vi "Data Sender.vi"() -> ()   [LabVIEW 2018]
uses:
  <vilib>/userdefined/High Color/IMAQdx.ctl
  <vilib>/DAQmx/read.llb/DAQmx Read (Analog 2D DBL NChan NSamp).vi
  <vilib>/DAQmx/miscellaneous.llb/DAQmx Fill In Error Info.vi
  <vilib>/vision/driver/NI_Vision_Acquisition_Software.lvlib
panel:
  in  "Stop 2":bool
  in  "Save Binary":bool
  in  "Save AVI":bool
  out "Image 3":T1(plugin-control)
  in  "Image Type":T2 items=["Grayscale (U8)", "Grayscale (I16)", "Grayscale (SGL)", "Complex (CSG)", "RGB (U32)", "HSL (U32)", "RGB (U64)", "Grayscale (U16)"]
  out "Frame Number Recorded":i32
  in  "number":i32
  in  "File Folder":path
  in  "Video Camera":T3 caption="Camera Name"
  # "Binary Video"
  # "AVI Video"
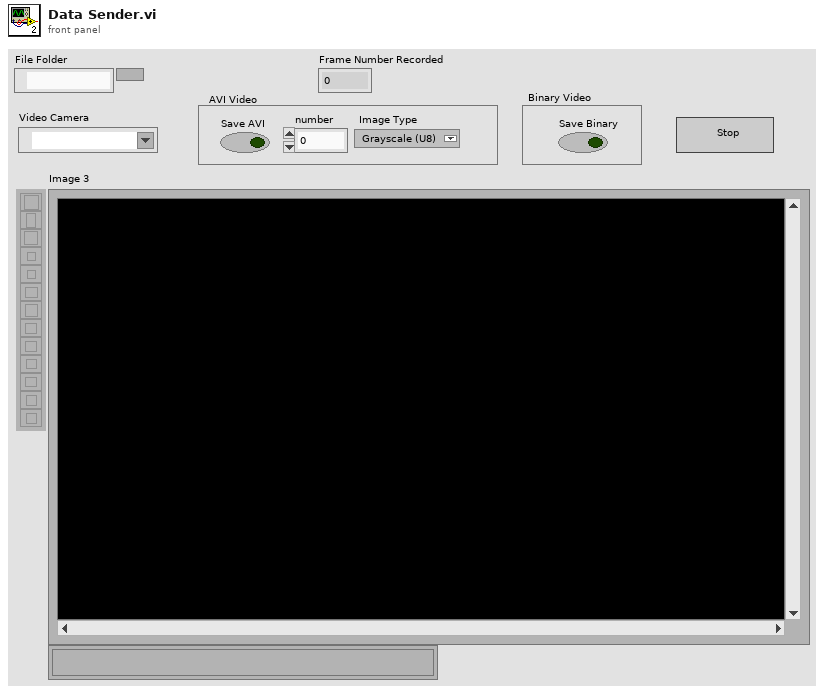
[diagram p1: front panel]
types:
  T1 = typedef "IMAQ Image.ctl" = refnum<image>
  T2 = typedef "Image Type" = u32
  T3 = typedef "IMAQdx.ctl" = refnum<k21>
  T4 = typedef "IMAQ AVI2 Refnum.ctl" = refnum<k20>
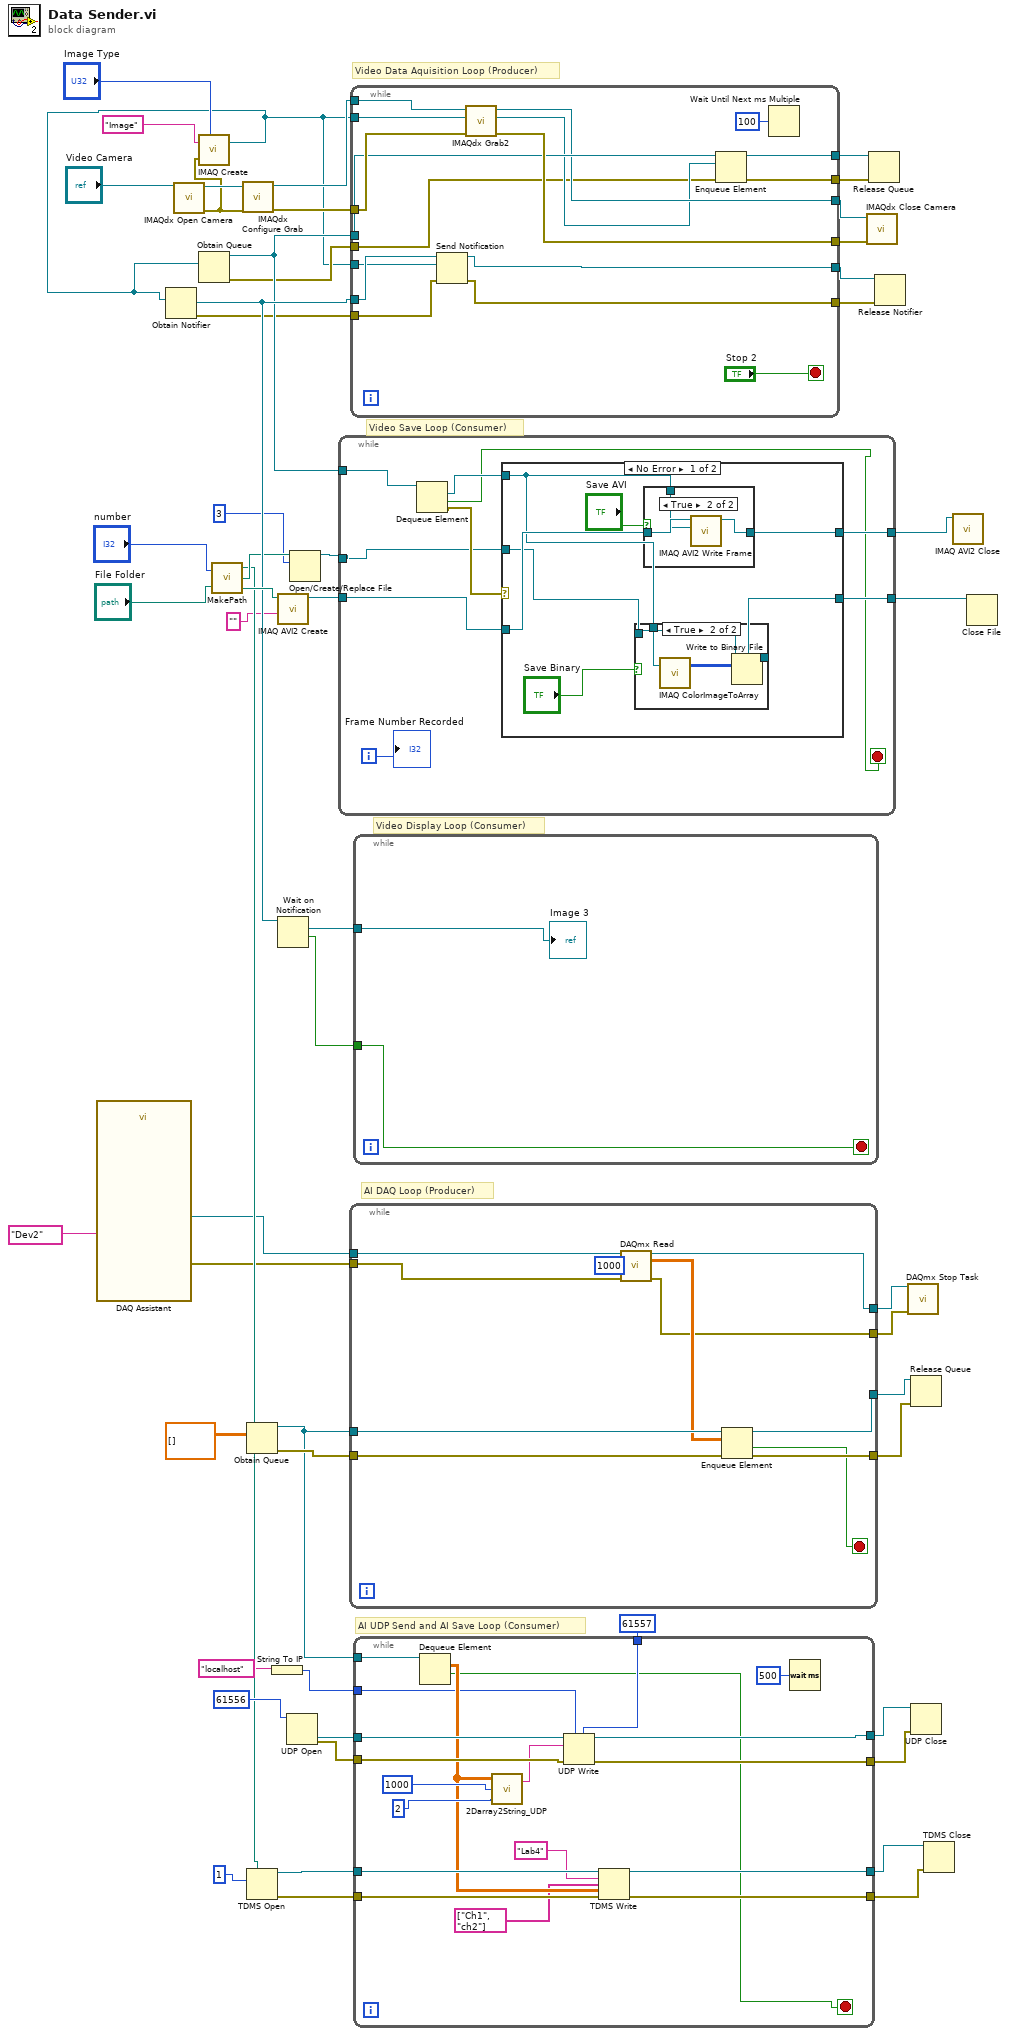
[diagram p0: block diagram]
diagram:
  # "AI UDP Send and AI Save Loop (Consumer)"
  # "AI DAQ Loop (Producer)"
  # "Video Display Loop (Consumer)"
  # "Video Save Loop (Consumer)"
  # "Video Data Aquisition Loop (Producer)"
  n1 = call "DAQ Assistant"("device name"=tag "Dev2") -> ("task out"=w7:refnum<k21>, "error out"=w6:errorcluster)  [unwired: 15 in, 2 out]
  n2 = call <vilib>:"IMAQdx Open Camera.vi"("Session In"="Video Camera") -> ("error out"=w45:errorcluster, "Session Out"=w53:T3)  [unwired: 9 in]
  n3 = call "IMAQ Create"("Image Name"="Image", "Image Type"="Image Type", "error in (no error)"=w45) -> ("New Image"=w27:T1)  [unwired: 2 in, 1 out]
  n4 = Obtain Notifier(notification data type=w27) -> (notifier out=w40:refnum<notifier>, error out=w32:errorcluster)  [unwired: 3 in, 1 out]
  n5 = Obtain Queue(element data type=w27) -> (queue out=w38:refnum<queue>, error out=w30:errorcluster)  [unwired: 4 in, 1 out]
  n6 = call "MakePath.vi"("Numeric"="number", "Path"="File Folder") -> ("TDMS"=w8:path, "BIN"=w35:path, "AVI"=w44:path)
  n7 = call <vilib>:"IMAQdx Configure Grab.vi"("error in"=w45, "Session In"=w53) -> ("error out"=w52:errorcluster, "Session Out"=w33:T3)  [unwired: 8 in]
  n8 = Obtain Queue(element data type=dbl[][] [] ("data")) -> (queue out=w11:refnum<queue>, error out=w22:errorcluster)  [unwired: 4 in, 1 out]
  n9 = TDMS Open(10:1, 11:w8) -> (0:w15:errorcluster, 3:w16:refnum<k34>)  [unwired: 5 in]
  n10 = String To IP(1:"localhost") -> (0:w2:u32)
  n11 = call "IMAQ AVI2 Create"("Codec"="", "AVI Path"=w44) -> ("AVI Refnum"=w43:T4)  [unwired: 8 in, 1 out]
  n12 = Wait on Notification(notifier=w40) -> (notification=w39:T1, timed out?=w9:bool)  [unwired: 3 in, 2 out]
  n13 = UDP Open(11:61556) -> (port=w20:refnum<k16>, 0:w21:errorcluster)  [unwired: 4 in, 1 out]
  n14 = Open/Create/Replace File(file path (use dialog)=w35, operation (0:open)=3) -> (refnum out=w36:refnum<file>)  [unwired: 4 in, 2 out]
  n15 = while {
    tunnel: w43 -> [w60]
    tunnel: w36 -> [w61]
    tunnel: [w59] -> w42
    tunnel: [w58] -> w41
    tunnel: w38 -> [w57]
    i -> [w62]
    stop <- w55 stop-if-true
    n16 = Dequeue Element(queue=w57) -> (element=w56:T1, timed out?=w55:bool, error out=w63:errorcluster)  [unwired: 2 in, 1 out]
    n17 = case shown="No Error" w63 {
      tunnel: w61 -> [w69 w80]
      tunnel: w60 -> [w70 w81]
      tunnel: [w68 w81] -> w59
      tunnel: [w67 w80] -> w58
      tunnel: w56 -> [w66 _]
      frame No Error {
        n18 = case shown="True" "Save Binary" {
          tunnel: w69 -> [w71 w75]
          tunnel: [w71 w74] -> w67
          tunnel: w66 -> [_ w73]
          frame False {
          }
          frame True {
            n19 = call "IMAQ ColorImageToArray"("Image"=w73) -> ("Image Pixels (U32)"=w72:u32[][])  [unwired: 3 in, 2 out]
            n20 = Write to Binary File(file (use dialog)=w75, data=w72) -> (refnum out=w74:refnum<file>)  [unwired: 4 in, 2 out]
          }
        }
        n21 = case shown="True" "Save AVI" {
          tunnel: w70 -> [w76 w79]
          tunnel: [w76 w78] -> w68
          tunnel: w66 -> [_ w77]
          frame False {
          }
          frame True {
            n22 = call "IMAQ AVI2 Write Frame"("Image"=w77, "AVI Refnum"=w79) -> ("AVI Refnum (duplicate)"=w78:T4)  [unwired: 7 in, 2 out]
          }
        }
      }
      frame Error {
      }
    }
    "Frame Number Recorded" <- w62
  }
  n23 = while {
    tunnel: w11 -> [w92]
    tunnel: [w86] -> w26
    tunnel: [w87] -> w25
    tunnel: [w91] -> w24
    tunnel: [w90] -> w23
    tunnel: w22 -> [w89]
    tunnel: w7 -> [w83]
    tunnel: w6 -> [w82]
    stop <- w85 stop-if-true
    n24 = call-poly <vilib>:"DAQmx Read.vi"("task/channels in"=w83, "number of samples per channel"=1000, "error in"=w82) -> ("task out"=w86:refnum<k21>, "data"=w88:dbl[][], "error out"=w87:errorcluster)  [unwired: 10 in]
    n25 = Enqueue Element(queue=w92, element=w88, error in (no error)=w89) -> (queue out=w91:refnum<queue>, timed out?=w85:bool, error out=w90:errorcluster)  [unwired: 1 in]
  }
  n26 = while {
    tunnel: w52 -> [w109]
    tunnel: [w108] -> w29
    tunnel: [w105] -> w51
    tunnel: w38 -> [w106]
    tunnel: [w107] -> w50
    tunnel: w40 -> [w95]
    tunnel: [w100] -> w48
    tunnel: w33 -> [w103]
    tunnel: w27 -> [w102]
    tunnel: w32 -> [w99]
    tunnel: [w98] -> w31
    tunnel: w30 -> [w97]
    tunnel: [w96] -> w28
    tunnel: w27 -> [w94]
    stop <- "Stop 2" stop-if-true
    n27 = Send Notification(notification=w94, notifier=w95, error in (no error)=w99) -> (notifier out=w100:refnum<notifier>, error out=w98:errorcluster)
    n28 = call <vilib>:"IMAQdx Grab2.vi"("error in"=w109, "Image In"=w102, "Session In"=w103) -> ("error out"=w108:errorcluster, "Image Out"=w104:T1, "Session Out"=w105:T3)  [unwired: 5 in, 1 out]
    n29 = Enqueue Element(queue=w106, element=w104, error in (no error)=w97) -> (queue out=w107:refnum<queue>, error out=w96:errorcluster)  [unwired: 1 in, 1 out]
    n30 = Wait Until Next ms Multiple(millisecond multiple=u32 100) -> ()  [unwired: 1 out]
  }
  n31 = while {
    tunnel: w39 -> [w111]
    tunnel: w9 -> [w110]
    stop <- w110 stop-if-true
    "Image 3" <- w111
  }
  n32 = while {
    tunnel: w21 -> [w130]
    tunnel: w20 -> [w129]
    tunnel: [w128] -> w19
    tunnel: [w127] -> w18
    tunnel: w16 -> [w126]
    tunnel: w15 -> [w125]
    tunnel: [w124] -> w14
    tunnel: [w114] -> w13
    tunnel: w11 -> [w123]
    tunnel: w2 -> [w116]
    tunnel: 61557 -> [w115]
    stop <- w112 stop-if-true
    n33 = Dequeue Element(queue=w123) -> (element=w120:dbl[][], timed out?=w112:bool)  [unwired: 2 in, 2 out]
    n34 = call "2Darray2String_UDP.vi"("NumOfCH"=2, "NumberOfSamples"=1000, "Waveform Graph"=w120) -> ("UDP_String"=w117:string)  [unwired: 1 out]
    n35 = UDP Write(address=w116, port or service name=w115, connection ID=w129, data in=w117, 8:w130) -> (error out=w127:errorcluster, 3:w128:refnum<k16>)  [unwired: 1 in]
    n36 = TDMS Write(0:w126, 5:"Lab4" ("group name in (Untitled)"), 7:string[] ["Ch1", "ch2"] ("channel name(s) in (Untitled)"), 9:w120, 11:w125) -> (4:w124:refnum<k34>, 15:w114:errorcluster)  [unwired: 1 in, 2 out]
    n37 = Wait (ms)(milliseconds to wait=u32 500) -> ()  [unwired: 1 out]
  }
  n38 = call <vilib>:"IMAQdx Close Camera.vi"("error in"=w29, "Session In"=w51) -> ()  [unwired: 9 in, 1 out]
  n39 = Release Queue(queue=w50, error in (no error)=w28) -> ()  [unwired: 1 in, 3 out]
  n40 = Release Notifier(notifier=w48, error in (no error)=w31) -> ()  [unwired: 1 in, 3 out]
  n41 = call <vilib>:"DAQmx Stop Task.vi"("task/channels in"=w26, "error in"=w25) -> ()  [unwired: 12 in, 2 out]
  n42 = Release Queue(queue=w24, error in (no error)=w23) -> ()  [unwired: 1 in, 3 out]
  n43 = UDP Close(connection ID=w19, 8:w18) -> ()  [unwired: 2 out]
  n44 = TDMS Close(8:w13, 11:w14) -> ()  [unwired: 2 out]
  n45 = call "IMAQ AVI2 Close"("AVI Refnum"=w42) -> ()  [unwired: 10 in, 1 out]
  n46 = Close File(refnum=w41) -> ()  [unwired: 1 in, 2 out]
